vi "Shutdown.vi"(8 "error in (no error)":errorcluster, 11 "VolatusCoreTask in":refnum<class "VolatusCoreTask.lvclass">) -> (0 "error out":errorcluster, 3 "VolatusCoreTask out":refnum<class "VolatusCoreTask.lvclass">)   [LabVIEW 2020, in "Volatus.lvlib" / "VolatusCoreTask.lvclass"]
uses:
  VolatusCoreTask.lvclass
  VolatusCoreTask.lvclass/VolatusCoreTask.ctl
  <vilib>/ActorFramework/Actor/Actor.lvclass
  <vilib>/ActorFramework/Stop Msg/Stop Msg.lvclass
  C:/dev/lv20CE/relink/lv-volatus/Volatus/Task/Task.lvclass
  C:/Program Files (x86)/National Instruments/LabVIEW 2020/vi.lib/ActorFramework/Actor/Actor.lvclass
  C:/dev/lv20CE/relink/lv-volatus/Volatus/APIRegistrationHandler/APIRegistrationHandler.lvclass
  C:/dev/lv20CE/relink/lv-volatus/Volatus/TaskStateHandler/TaskStateHandler.lvclass
  C:/dev/lv20CE/relink/lv-volatus/Volatus/VectoMessageHandler/VectoMessageHandler.lvclass
  C:/dev/lv20CE/relink/lv-volatus/Volatus/VolatusCoreTask/VolatusCoreTask.lvclass
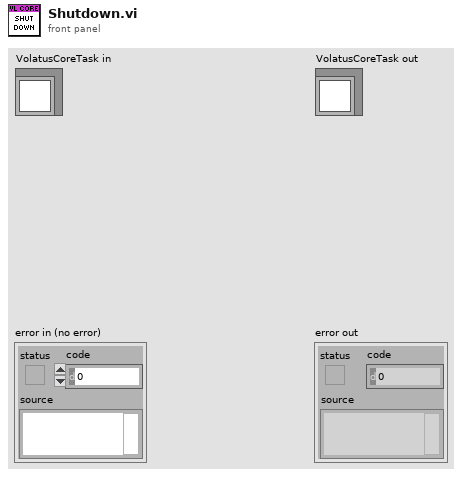
[diagram p1: front panel]
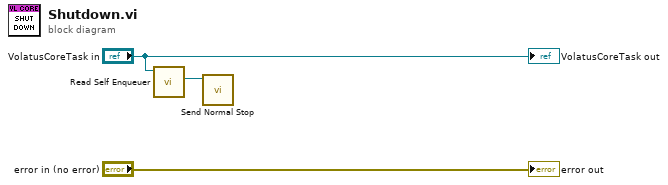
[diagram p0: block diagram]
diagram:
  n1 = call <vilib>:"Read Self Enqueuer.vi"("Actor"="VolatusCoreTask in") -> ("Self Enqueuer"=w1:refnum<class "Message Enqueuer.lvclass">)  [unwired: 10 in]
  n2 = call <vilib>:"Send Normal Stop.vi"("Message Enqueuer"=w1) -> ()  [unwired: 10 in, 1 out]
  "error out" <- "error in (no error)"
  "VolatusCoreTask out" <- "VolatusCoreTask in"
